vi "TCP Server.vi"() -> ()   [LabVIEW 2014]
panel:
  in  "정지":bool
  out "웨이브폼 그래프":dbl[](graph)
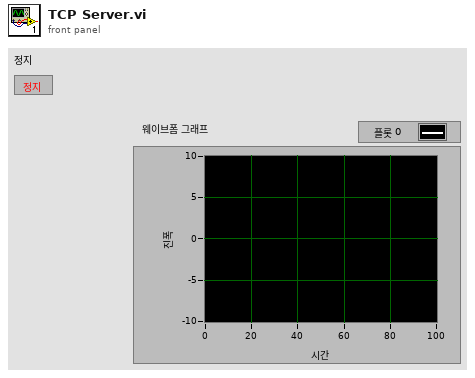
[diagram p1: front panel]
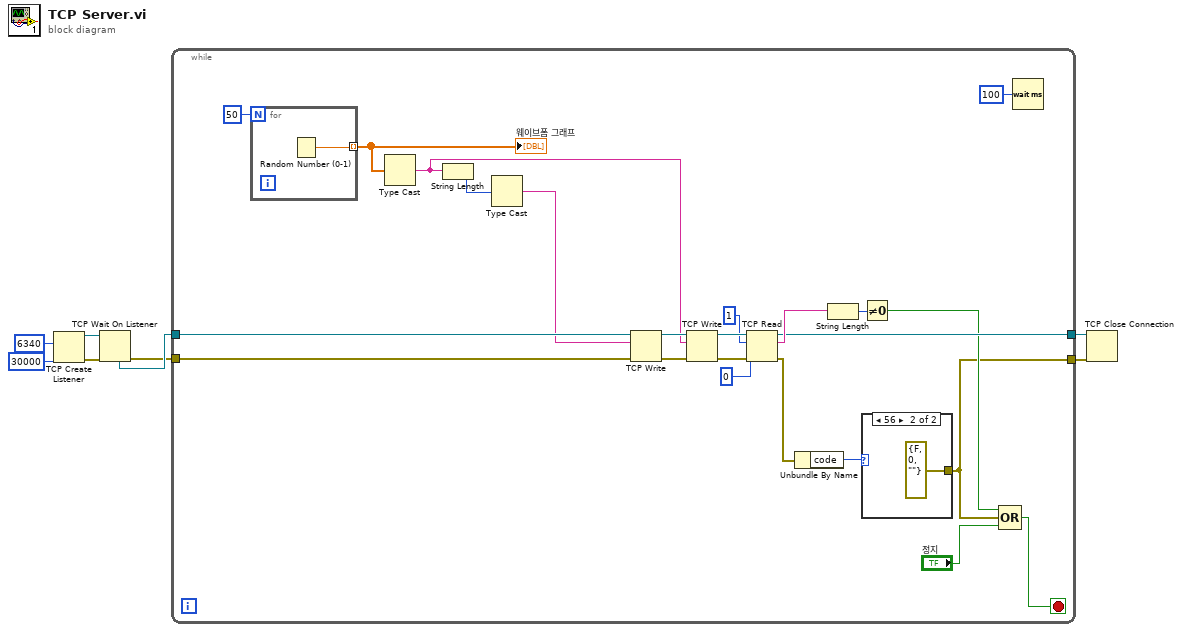
[diagram p0: block diagram]
diagram:
  n1 = TCP Create Listener(9:30000 ("타임아웃 ms (25000)"), 10:u16 6340 ("포트")) -> (0:w8:errorcluster, 3:w7:refnum<k5>)  [unwired: 3 in, 1 out]
  n2 = TCP Wait On Listener(8:w8, 11:w7) -> (0:w3:errorcluster, 4:w4:refnum<k5>)  [unwired: 2 in, 3 out]
  n3 = while {
    tunnel: w4 -> [w28]
    tunnel: w3 -> [w26]
    tunnel: [w17] -> w1
    tunnel: [w12] -> w2
    stop <- w11 stop-if-true
    n4 = for {
      N: 50 -> [_]
      tunnel: [w33] -> w30 mode=indexing
      n5 = Random Number (0-1)() -> (number: 0 to 1=w33:dbl)
    }
    "웨이브폼 그래프" <- w30
    n6 = Type Cast(x=w30) -> (*(type *) &x=w23:string)  [unwired: 1 in]
    n7 = String Length(string=w23) -> (length=w29:i32)
    n8 = Type Cast(x=w29) -> (*(type *) &x=w27:string)  [unwired: 1 in]
    n9 = TCP Write(connection ID=w28, data in=w27, error in (no error)=w26) -> (connection ID out=w24:refnum<k5>, error out=w25:errorcluster)  [unwired: 1 in, 1 out]
    n10 = TCP Write(connection ID=w24, data in=w23, error in (no error)=w25) -> (connection ID out=w22:refnum<k5>, error out=w21:errorcluster)  [unwired: 1 in, 1 out]
    n11 = TCP Read(connection ID=w22, bytes to read=1 ("읽을 바이트"), error in (no error)=w21, 9:0 ("타임아웃 ms (25000)")) -> (connection ID out=w17:refnum<k5>, data out=w18:string, error out=w14:errorcluster)  [unwired: 1 in]
    n12 = Unbundle By Name(w14) -> ("code"=w13:i32)
    n13 = String Length(string=w18) -> (length=w16:i32)
    n14 = Not Equal To 0?(x=w16) -> (x != 0?=w15:bool)
    n15 = case shown="56" w13 {
      tunnel: [_ errorcluster {"status"=FALSE, "code"=0, "source"=""} ("에러 상수")] -> w12
      frame 0, Default {
      }
      frame 56 {
      }
    }
    n16 = Compound Arithmetic op=OR(w15, w12, "정지") -> (w11:bool)
    n17 = Wait (ms)(milliseconds to wait=u32 100 ("대기 시간(ms)")) -> ()  [unwired: 1 out]
  }
  n18 = TCP Close Connection(connection ID=w1, error in (no error)=w2) -> ()  [unwired: 1 in, 2 out]
